vi "PRINT OLD RECEIPT.vi"(11 "REFERENCES":T1) -> ()   [LabVIEW 2019]
uses:
  Controls/References Cluster.ctl
  Controls/Custom Calendar/Custom Calendar.xctl
  <vilib>/addons/database/Auxilliary.llb/DB Tools Cursor Type.ctl
  Controls/Table Data Types/PSC Sales Data Type.ctl
  <vilib>/Utility/NIReport.llb/Report Type.ctl
  <vilib>/addons/database/Connection.llb/DB Tools Open Connec (String).vi
  <vilib>/addons/database/Connection.llb/Conn Execute.vi
  <vilib>/addons/database/Recordset.llb/Rec Fetch Recordset Data (R).vi
  <vilib>/addons/database/Recordset.llb/Rec Destroy - Connection.vi
  <vilib>/Utility/NIReport.llb/Append Report Text (str wrap).vi
  <vilib>/Utility/NIReport.llb/Append Text Table to Report (wrap).vi
  <vilib>/addons/database/_DB Variant To Data/Database Variant To Data.xnode
  <vilib>/Utility/NIReport.llb/NI_report.lvclass
  <vilib>/addons/database/NI_Database_API.lvlib
  <vilib>/Utility/NIReport.llb/NI_ReportGenerationCore.lvlib
  <vilib>/Utility/NIReport.llb/Word/NI_Word.lvclass
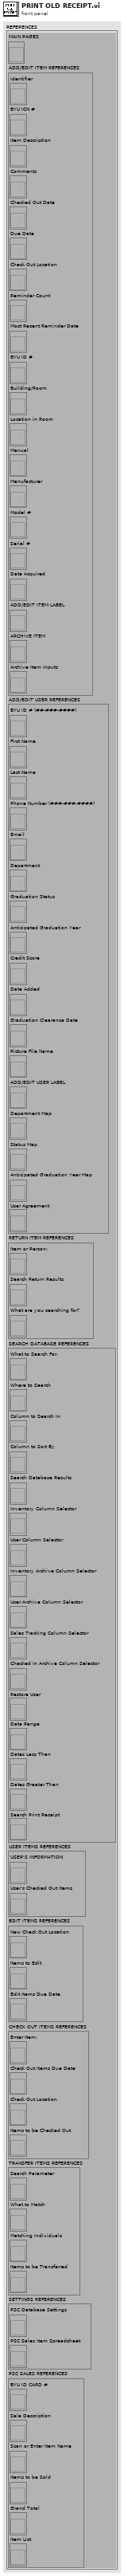
[diagram p1: front panel]
types:
  T1 = typedef "References Cluster.ctl" = cluster{"MAIN PAGES":refnum<vi>, "ADD/EDIT ITEM REFERENCES":cluster{"Identifier":refnum<vi>, "BYU ICN #":refnum<vi>, "Item Description":refnum<vi>, "Comments":refnum<vi>, "Checked Out Date":refnum<vi>, "Due Date":refnum<vi>, "Check Out Location":refnum<vi>, "Reminder Count":refnum<vi>, "Most Recent Reminder Date":refnum<vi>, "BYU ID #":refnum<vi>, "Building/Room":refnum<vi>, "Location in Room":refnum<vi>, "Manual":refnum<vi>, "Manufacturer":refnum<vi>, "Model #":refnum<vi>, "Serial #":refnum<vi>, "Date Acquired":refnum<vi>, "ADD/EDIT ITEM LABEL":refnum<vi>, "ARCHIVE ITEM":refnum<vi>, "Archive Item Inputs":refnum<vi>}, "ADD/EDIT USER REFERENCES":cluster{"BYU ID # (##-###-####)":refnum<vi>, "First Name":refnum<vi>, "Last Name":refnum<vi>, "Phone Number (###-###-####)":refnum<vi>, "Email":refnum<vi>, "Department":refnum<vi>, "Graduation Status":refnum<vi>, "Anticipated Graduation Year":refnum<vi>, "Credit Score":refnum<vi>, "Date Added":refnum<vi>, "Graduation Clearance Date":refnum<vi>, "Picture File Name":refnum<vi>, "ADD/EDIT USER LABEL":refnum<vi>, "Department Map":refnum<vi>, "Status Map":refnum<vi>, "Anticipated Graduation Year Map":refnum<vi>, "User Agreement":refnum<vi>}, "RETURN ITEM REFERENCES":cluster{"Item or Person:":refnum<vi>, "Search Return Results":refnum<vi>, "What are you searching for?":refnum<vi>}, "SEARCH DATABASE REFERENCES":cluster{"What to Search For:":refnum<vi>, "Where to Search":refnum<vi>, "Column to Search In":refnum<vi>, "Column to Sort By":refnum<vi>, "Search Database Results":refnum<vi>, "Inventory Column Selector":refnum<vi>, "User Column Selector":refnum<vi>, "Inventory Archive Column Selector":refnum<vi>, "User Archive Column Selector":refnum<vi>, "Sales Tracking Column Selector":refnum<vi>, "Checked In Archive Column Selector":refnum<vi>, "Restore User":refnum<vi>, "Date Range":refnum<vi>, "Dates Less Than":refnum<vi>, "Dates Greater Than":refnum<vi>, "Search Print Receipt":refnum<vi>}, "USER ITEMS REFERENCES":cluster{"USER'S INFORMATION":refnum<vi>, "User's Checked Out Items":refnum<vi>}, "EDIT ITEMS REFERENCES":cluster{"New Check Out Location":refnum<vi>, "Items to Edit":refnum<vi>, "Edit Items Due Date":refnum<vi>}, "CHECK OUT ITEMS REFERENCES":cluster{"Enter Item:":refnum<vi>, "Check Out Items Due Date":refnum<vi>, "Check Out Location":refnum<vi>, "Items to be Checked Out":refnum<vi>}, "TRANSFER ITEMS REFERENCES":cluster{"Search Parameter":refnum<vi>, "What to Match":refnum<vi>, "Matching Individuals":refnum<vi>, "Items to be Transferred":refnum<vi>}, "SETTINGS REFERENCES":cluster{"PSC Database Settings":refnum<vi>, "PSC Sales Item Spreadsheet":refnum<vi>}, "PSC SALES REFERENCES":cluster{"BYU ID CARD #":refnum<vi>, "Sale Description":refnum<vi>, "Scan or Enter Item Name":refnum<vi>, "Items to be Sold":refnum<vi>, "Grand Total":refnum<vi>, "Item List":refnum<vi>}}
  T2 = cluster{"What to Search For:":refnum<vi>, "Where to Search":refnum<vi>, "Column to Search In":refnum<vi>, "Column to Sort By":refnum<vi>, "Search Database Results":refnum<vi>, "Inventory Column Selector":refnum<vi>, "User Column Selector":refnum<vi>, "Inventory Archive Column Selector":refnum<vi>, "User Archive Column Selector":refnum<vi>, "Sales Tracking Column Selector":refnum<vi>, "Checked In Archive Column Selector":refnum<vi>, "Restore User":refnum<vi>, "Date Range":refnum<vi>, "Dates Less Than":refnum<vi>, "Dates Greater Than":refnum<vi>, "Search Print Receipt":refnum<vi>}
  T3 = typedef "PSC Sales Data Type.ctl" = cluster{"SALE ID #":string, "BYU ID CARD #":string, "Sale Description":string, "Grand Total":string, "Sale Date":string, "Item Description":string, "Item Quantity":string, "Item Unit Price":string, "Item Total Price":string, "Sale Semester":string}
  T4 = typedef "NI_Database_API.lvlib/DB Tools Cursor Type.ctl" = enum16{"forward-only", "keyset", "dynamic", "static"}
  T5 = cluster{"position (excel)":cluster{"row":i32, "column":i32}, "name (excel)":string, "bookmark (word)":string}
  T6 = typedef "NI_ReportGenerationCore.lvlib/Report Type.ctl" = enum16{"HTML", "Word", "Excel"}
  T7 = enum16{"maximized", "minimized", "normal", "no change"}
  T8 = typedef "NI_Database_API.lvlib/Conn ObjectReference.ctl" = refnum<k1>
  T9 = typedef "NI_Database_API.lvlib/Rec ObjectReference.ctl" = refnum<k1>
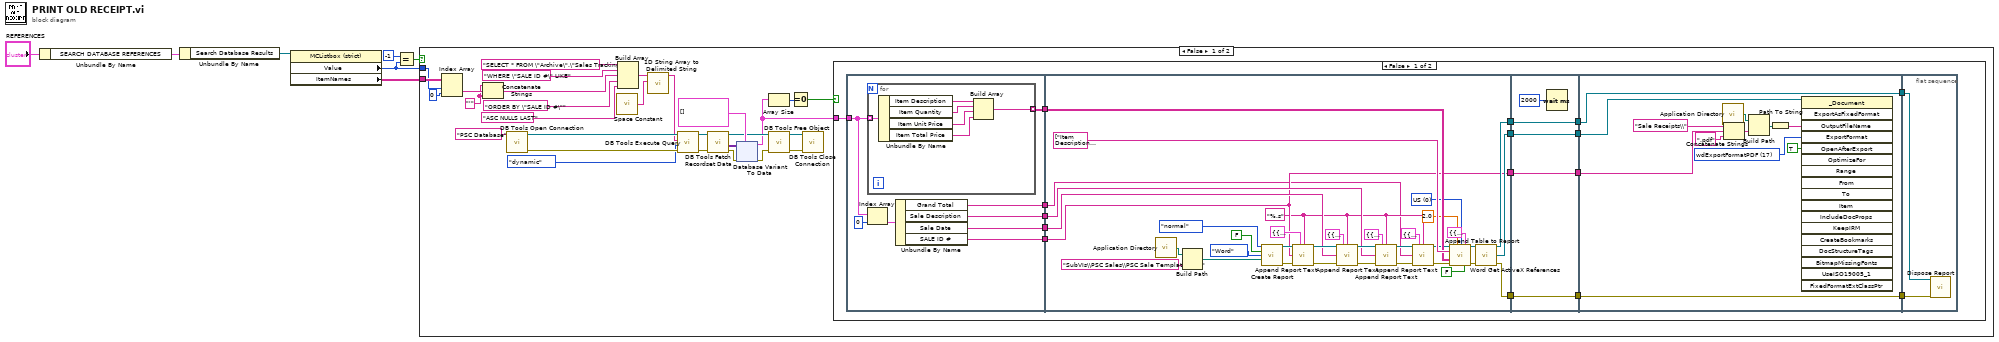
[diagram p0: block diagram]
diagram:
  n1 = Unbundle By Name("REFERENCES") -> ("SEARCH DATABASE REFERENCES"=w6:T2)
  n2 = Unbundle By Name(w6) -> ("Search Database Results"=w5:refnum<vi>)
  n3 = property class="MCListbox (strict)"(reference=w5) -> ("Value"=w2:i32, "ItemNames"=w1:string[][])  [unwired: 1 in, 2 out]
  n4 = Equal?(x=-1, y=w2) -> (x = y?=w3:bool)
  n5 = case shown="False" w3 {
    tunnel: w2 -> [w35 _]
    tunnel: w1 -> [w36 _]
    frame False {
      w28 = "'" ("string")
      n6 = Index Array(array=w36, index (row)=w35, index (col)=0 ("disabled index (col)")) -> (element=w29:string)
      n7 = Concatenate Strings(w28, w29, w28) -> (w26:string)
      n8 = call-poly <vilib>:"DB Tools Open Connection.vi"("connection information"="PSC Database" ("string")) -> ("error out"=w23:errorcluster, "connection reference"=w24:T8)  [unwired: 7 in]
      n9 = call <vilib>:"Space Constant.vi"() -> ("String"=w32:string)
      n10 = Build Array("SELECT * FROM \"Archive\".\"Sales Tracking\"" ("string"), "WHERE \"SALE ID #\" LIKE" ("string"), w26, "ORDER BY \"SALE ID #\"" ("string"), "ASC NULLS LAST" ("string")) -> (w33:string[])
      n11 = call <vilib>:"1D String Array to Delimited String.vi"("delimiter"=w32, "string array"=w33) -> ("delimited string"=w22:string)  [unwired: 9 in]
      n12 = call-poly <vilib>:"DB Tools Execute Query.vi"("error in (no error)"=w23, "cursor type"=DB_Tools_Cursor_Type."dynamic", "SQL query"=w22, "connection reference"=w24) -> ("error out"=w19:errorcluster, "recordset reference"=w20:T9)  [unwired: 4 in]
      n13 = call-poly <vilib>:"DB Tools Fetch Recordset Data.vi"("error in (no error)"=w19, "recordset reference"=w20) -> ("error out"=w16:errorcluster, "recordset data"=w18:variant[][], "recordset reference out"=w14:T9)  [unwired: 3 in]
      n14 = xnode "Database Variant To Data"("database variant"=w18, "error in (no error)"=w16, "type"=T3[] [] ("Array")) -> ("data"=w9:T3[], "error out"=w13:errorcluster)
      n15 = Array Size(array=w9) -> (size(s)=w15:i32)
      n16 = call-poly <vilib>:"DB Tools Free Object.vi"("error in (no error)"=w13, "recordset reference"=w14) -> ("error out"=w11:errorcluster, "connection reference"=w12:T8)  [unwired: 8 in]
      n17 = Equal To 0?(x=w15) -> (x = 0?=w10:bool)
      n18 = call <vilib>:"DB Tools Close Connection.vi"("error in (no error)"=w11, "connection reference"=w12) -> ()  [unwired: 5 in, 1 out]
      n19 = case shown="False" w10 {
        tunnel: w9 -> [w52 _]
        frame False {
          n20 = flat-sequence {
            tunnel: w52 -> [w60]
            tunnel: [w57] -> w51
            tunnel: [w56] -> w50
            tunnel: [w55] -> w49
            tunnel: [w54] -> w48
            tunnel: [w53] -> w37
            tunnel: w51 -> [w77]
            tunnel: w50 -> [w84]
            tunnel: w49 -> [w83]
            tunnel: w48 -> [w81]
            tunnel: [w80] -> w47
            tunnel: [w79] -> w46
            tunnel: [w78] -> w43
            tunnel: [w77] -> w40
            tunnel: w37 -> [w70]
            tunnel: w47 -> [w106]
            tunnel: w46 -> [w105]
            tunnel: [w106] -> w45
            tunnel: [w105] -> w44
            tunnel: w43 -> [w104]
            tunnel: [w104] -> w42
            tunnel: [w103] -> w41
            tunnel: w40 -> [w103]
            tunnel: w45 -> [w110]
            tunnel: w44 -> [w109]
            tunnel: w42 -> [w108]
            tunnel: w41 -> [w111]
            tunnel: [w110] -> w39
            tunnel: [w108] -> w38
            tunnel: w39 -> [w121]
            tunnel: w38 -> [w120]
            frame #0 {
              n21 = for {
                tunnel: w60 -> [w66] mode=indexing
                tunnel: [w61] -> w54 mode=indexing
                n22 = Unbundle By Name(w66) -> ("Item Description"=w65:string, "Item Quantity"=w64:string, "Item Unit Price"=w63:string, "Item Total Price"=w62:string)
                n23 = Build Array(w65, w64, w63, w62) -> (w61:string[])
              }
              n24 = Index Array(array=w60, index=0) -> (element=w58:T3)
              n25 = Unbundle By Name(w58) -> ("Grand Total"=w53:string, "Sale Description"=w55:string, "Sale Date"=w56:string, "SALE ID #"=w57:string)
            }
            frame #1 {
              w69 = u16 0 items=["US", "Metric", "Default"] ("measurement system")
              w72 = "%.s" ("format string (%.3f)")
              n26 = call <vilib>:"Application Directory.vi"() -> ("Application Directory"=w101:path)
              n27 = Build Path(base path=w101, name or relative path="SubVIs\\PSC Sales\\PSC Sale Template.dotx") -> (appended path=w102:path)
              n28 = call <vilib>:"Create Report.vi"("window state (normal)"=T7."normal", "display alerts? (F)"=FALSE, "report type"=Report_Type."Word", "template (empty)"=w102) -> ("report out"=w93:refnum<class "NI_report.lvclass">, "error out"=w94:errorcluster)  [unwired: 10 in]
              n29 = call-poly <vilib>:"Append Report Text.vi"("report in"=w93, "MS Office parameters"=T5 {"position (excel)"={"row"=0, "column"=0}, "name (excel)"="", "bookmark (word)"="Sale_ID"}, "format string (%.3f)"=w72, "text"=w77, "error in (no error)"=w94) -> ("report out"=w95:refnum<class "NI_report.lvclass">, "error out"=w96:errorcluster)  [unwired: 7 in, 2 out]
              n30 = call-poly <vilib>:"Append Report Text.vi"("report in"=w95, "MS Office parameters"=T5 {"position (excel)"={"row"=0, "column"=0}, "name (excel)"="", "bookmark (word)"="Sale_Date"}, "format string (%.3f)"=w72, "text"=w84, "error in (no error)"=w96) -> ("report out"=w99:refnum<class "NI_report.lvclass">, "error out"=w100:errorcluster)  [unwired: 7 in, 2 out]
              n31 = call-poly <vilib>:"Append Report Text.vi"("report in"=w99, "MS Office parameters"=T5 {"position (excel)"={"row"=0, "column"=0}, "name (excel)"="", "bookmark (word)"="Sale_Description"}, "format string (%.3f)"=w72, "text"=w83, "error in (no error)"=w100) -> ("report out"=w76:refnum<class "NI_report.lvclass">, "error out"=w75:errorcluster)  [unwired: 7 in, 2 out]
              n32 = call-poly <vilib>:"Append Report Text.vi"("report in"=w76, "MS Office parameters"=T5 {"position (excel)"={"row"=0, "column"=0}, "name (excel)"="", "bookmark (word)"="Sale_Grand_Total"}, "format string (%.3f)"=w72, "text"=w70, "error in (no error)"=w75) -> ("report out"=w73:refnum<class "NI_report.lvclass">, "error out"=w74:errorcluster)  [unwired: 7 in, 2 out]
              n33 = call-poly <vilib>:"Append Table to Report.vi"("report in"=w73, "column width (1)"=2.0, "measurement system"=w69, "MS Office parameters"=T5 {"position (excel)"={"row"=0, "column"=0}, "name (excel)"="", "bookmark (word)"="Sale_Items"}, "column headers"=string[] ["Item Description", "Item Quantity", "Item Unit Price", "Item Total Price"], "text data"=w81, "error in (no error)"=w74, "show grid lines (YES)"=FALSE) -> ("report out"=w97:refnum<class "NI_report.lvclass">, "error out"=w98:errorcluster)  [unwired: 4 in, 2 out]
              n34 = call <vilib>:"Word Get ActiveX References.vi"("report in"=w97, "error in (no error)"=w98) -> ("report out"=w80:refnum<class "NI_report.lvclass">, "Word._Document"=w79:refnum<k7>, "error out"=w78:errorcluster)  [unwired: 7 in, 4 out]
            }
            frame #2 {
              n35 = Wait (ms)(milliseconds to wait=u32 2000) -> ()  [unwired: 1 out]
            }
            frame #3 {
              w113 = 17 items=["wdExportFormatPDF"=17, "wdExportFormatXPS"=18] ("ExportFormat")
              n36 = call <vilib>:"Application Directory.vi"() -> ("Application Directory"=w116:path)
              n37 = Concatenate Strings("Sale Receipts\\" ("name or relative path"), w111, ".pdf" ("name or relative path")) -> (w117:string)
              n38 = Build Path(base path=w116, name or relative path=w117) -> (appended path=w118:path)
              n39 = Path To String(path=w118) -> (string=w119:string)
              n40 = invoke class="_Document" method="ExportAsFixedFormat"(reference=w109, "OutputFileName"=w119, "ExportFormat"=w113, "OpenAfterExport"=TRUE) -> ()  [unwired: 14 in, 18 out]
            }
            frame #4 {
              n41 = call-dynamic "Dispose Report.vi"("report in"=w121, "error in (no error)"=w120) -> ()  [unwired: 13 in, 1 out]
            }
          }
        }
        frame True {
        }
      }
    }
    frame True {
    }
  }
